vi "MintDAQ.vi"() -> ()   [LabVIEW 2016]
panel:
  in  "Freq":dbl=0.01
  in  "Amplitude 2":dbl
  in  "Amplitude":dbl
  in  "Freq":dbl=0.03
  in  "Write Rate":dbl=10.0 caption="dt"
  in  "Sampling Rate":dbl=40000.0
  in  "Buffer Size":i32=2000
  in  "Write":bool
  in  "?":T1(tab)=enum."Feedback"
  out "Autocollimator":dynamicdata(graph)=[{"t0"=timestamp(3581195496.5418625 s since 1904-01-01), "dt"=0.001, "Y"=[3.3748341722363353, 3.3776633625283514, 3.37797401320521, 3.3775669552805136, 3.3771035700077543, 3.3768751556826606, 3.376331438110049, 3.3762235118309984, 3.3790075255607244, 3.376298514761084, 3.3752552067778043, 3.376255087955073, 3.377024337467859, 3.377016265489406, 3.3768109764991143, 3.377772600659941, 3.3750167885038906, 3.3758342740501286, 3.3778386645680794, 3.377603931037596, 3.3773015918402085, 3.377296761916378, 3.377247926722811, 3.37593401556452, 3.3774822825090043, 3.3787107942105887, 3.376029554612824, 3.376047566746657, 3.376884514809987, 3.377298833130131, 3.3776098386367988, 3.37785651466396, 3.378069066780402, 3.3750767036010347, 3.377711191620555, 3.3788531793882703, 3.37852043613071, 3.378316912955789, 3.3779787548920632, 3.378261441737476, 3.3769786144398255, 3.3793285877009565, 3.378617996670578, 3.3764510415055766, 3.3768974602491557, 3.377733875773734, 3.377895089879731, 3.377746964024869, 3.378223767761222, 3.3771328113007395], "attributes"=variant("NI_ChannelName"=variant(string "Voltage_0 (Resampled)"), "NI_OriginalChannelName"=variant(string "Voltage_0"), "NI_UnitDescription"=variant(string "Volts"))}, {"t0"=timestamp(3581195496.5418625 s since 1904-01-01), "dt"=0.001, "Y"=[-2.0834369730605644, -2.0819321459746876, -2.0815308696350567, -2.082042347246933, -2.082466743846781, -2.082543042435832, -2.0827169780126265, -2.082885379693655, -2.080652839627904, -2.0814165804978457, -2.0830704383386687, -2.0833234560752936, -2.082983892721974, -2.0825139979157505, -2.082384163355347, -2.0813173776580993, -2.0827868935770524, -2.0834134790149905, -2.081433686965862, -2.081283686189381, -2.082151524207096, -2.082631712746277, -2.082526422863312, -2.082716175637639, -2.082090913848439, -2.080153207335917, -2.081799074668808, -2.0828669505009736, -2.082318511827896, -2.081803388234694, -2.081634121622563, -2.081400526460551, -2.080924953428108, -2.082794281679033, -2.0818087503052656, -2.080747192813816, -2.0808949294383616, -2.081554802023675, -2.081683750116512, -2.0816670043945638, -2.082051426671936, -2.0805717294034096, -2.079922992538738, -2.081701961823228, -2.082161220322588, -2.0816213289100975, -2.0813481659597706, -2.0809482340093424, -2.080058560613854, -2.08051520256095], "attributes"=variant("NI_ChannelName"=variant(string "Voltage_1 (Resampled)"), "NI_OriginalChannelName"=variant(string "Voltage_1"), "NI_UnitDescription"=variant(string "Volts"))}, {"t0"=timestamp(3581195496.5418625 s since 1904-01-01), "dt"=0.001, "Y"=[3.3920512615889953, 3.3949128153687473, 3.3955558463709457, 3.3949822866205603, 3.3944043177259724, 3.394248244026162, 3.3936132739947547, 3.393681652979987, 3.396403586319937, 3.3936103172767687, 3.3923165107027082, 3.393375095157017, 3.3944467686804276, 3.3945298904876613, 3.394206680532547, 3.395118492820506, 3.3923967067110294, 3.393226765021611, 3.395338486732797, 3.3951997197019326, 3.39470966390894, 3.3946116821482164, 3.3948381609352896, 3.393475746046146, 3.395065077505499, 3.3961215980661974, 3.393416269199552, 3.393221438439225, 3.394214058418473, 3.3947867354978474, 3.39488924630533, 3.3953627275736626, 3.3952376332484664, 3.3923657648357612, 3.395027357033787, 3.396204609534961, 3.396065231694474, 3.395684684123652, 3.3954015147584964, 3.395557924959077, 3.394371246663519, 3.3966569176530097, 3.3957795238341366, 3.3936416739636406, 3.394088238066653, 3.394798352283088, 3.3951686004824486, 3.3950579729554087, 3.3957615999214954, 3.394260081617193], "attributes"=variant("NI_ChannelName"=variant(string "Voltage_2 (Resampled)"), "NI_OriginalChannelName"=variant(string "Voltage_2"), "NI_UnitDescription"=variant(string "Volts"))}, {"t0"=timestamp(3581195496.5418625 s since 1904-01-01), "dt"=0.001, "Y"=[-4.704546009666462, -4.7034172877833775, -4.702890947722384, -4.703542130524446, -4.703923265813428, -4.704021939575232, -4.703693488617615, -4.704025410027072, -4.702148224679809, -4.702052254209579, -4.703534587738418, -4.703962279465137, -4.703948009827787, -4.703470533679648, -4.703105555572077, -4.702091625546342, -4.702915333730992, -4.70395319557882, -4.702507570272585, -4.702193733835325, -4.702668184050766, -4.703115504299192, -4.70302121431319, -4.702854412488044, -4.702826487004598, -4.700608325540924, -4.701635969066888, -4.703172652877774, -4.702721955144197, -4.702259181304256, -4.701769735302749, -4.702025515044418, -4.701073609491946, -4.702417864320141, -4.7023704513299, -4.701403031144604, -4.701670663349241, -4.702326994974521, -4.702301569985744, -4.702431205539657, -4.702584562170047, -4.701553485457985, -4.7001882132184445, -4.701730869681846, -4.702741761914817, -4.702399160645309, -4.702126691528818, -4.701683926466696, -4.701055859883961, -4.701163846839676], "attributes"=variant("NI_ChannelName"=variant(string "Voltage_3 (Resampled)"), "NI_OriginalChannelName"=variant(string "Voltage_3"), "NI_UnitDescription"=variant(string "Volts"))}]
  out "Interferometer":dynamicdata(graph)=[{"t0"=timestamp(3581195496.558861 s since 1904-01-01), "dt"=0.001, "Y"=[2.5754216942498864, 2.5742770760564575, 2.5752864512365665, 2.5755975336972146, 2.5764982112217156, 2.578020182032285, 2.5787188766928537, 2.578606033584902, 2.579588876887395, 2.5813718560222414, 2.5824290269137053, 2.5833332167546144, 2.584973605142916, 2.5865313596086486, 2.5867840974371945, 2.5874262183925896, 2.5883498262197056, 2.5884123817913567, 2.5880556867115208, 2.588476459648385, 2.5890038740074224, 2.590149046746964, 2.590527470266104, 2.5908797553704233, 2.5908021249703337, 2.5911027120717267, 2.5906961773826267, 2.5906389426042766, 2.5910755741104285, 2.5900107369525407, 2.588926999990385, 2.5871153489787506, 2.5858600365775013, 2.583231765079389, 2.5812393863898278, 2.57896258373196, 2.5773304396580587, 2.5750683414591737, 2.5742551919858183, 2.573192991734795, 2.5716328992763873, 2.57007305058364, 2.568897523403074, 2.5678238474894224, 2.5667978328234895, 2.567077680460652, 2.5667571629855264, 2.5660656544367746, 2.5656740216609126, 2.565405291450495], "attributes"=variant("NI_ChannelName"=variant(string "Voltage_0 (Resampled)"), "NI_OriginalChannelName"=variant(string "Voltage_0"), "NI_UnitDescription"=variant(string "Volts"))}, {"t0"=timestamp(3581195496.558861 s since 1904-01-01), "dt"=0.001, "Y"=[1.2793515572809446, 1.285498354667561, 1.285530841442421, 1.2866454157673533, 1.2869733309979952, 1.2847744418721374, 1.2839067641968223, 1.2851830164941183, 1.2832161133825573, 1.279361456728847, 1.2759169068675607, 1.2741532340418997, 1.2698705062094546, 1.2653216768729953, 1.264148206169354, 1.2617013703491549, 1.2588960289321576, 1.2573198229314126, 1.2586716578972597, 1.2561926025230898, 1.2542066243656944, 1.2503531667795282, 1.2484903412768558, 1.2474317144212412, 1.2463530521075994, 1.245232527609533, 1.245115686074537, 1.2441214009515857, 1.241348303995827, 1.2429377222051292, 1.2445254511305113, 1.2472626848196695, 1.2486097094585318, 1.2526354072563082, 1.2550193843337556, 1.2578768598051189, 1.2589034076207384, 1.2608772152092518, 1.2596400197842403, 1.2585228801854373, 1.259170816804813, 1.2607258750064372, 1.2614748165179137, 1.2624939000744886, 1.2631031863313682, 1.2612009551189116, 1.2603436196192965, 1.2612488256841587, 1.2611557894880032, 1.260442702752587], "attributes"=variant("NI_ChannelName"=variant(string "Voltage_1 (Resampled)"), "NI_OriginalChannelName"=variant(string "Voltage_1"), "NI_UnitDescription"=variant(string "Volts"))}]
  out "Interferometer Angle":dynamicdata(graph)=[{"t0"=timestamp(3581195496.558873 s since 1904-01-01), "dt"=0.001, "Y"=[1.279385757759777, 1.2855094923223165, 1.2855542287511086, 1.2867099167763918, 1.286990419041426, 1.2847176486281568, 1.2838809934099638, 1.2851425707064237, 1.283210596160443, 1.2793465166695555, 1.2759426302074155, 1.274074922473625, 1.2697739936917296, 1.2652325471941344, 1.2641815410790656, 1.2617045191057616, 1.258894905178912, 1.2572982837418094, 1.2586022040497762, 1.2561475450207342, 1.254186491101226, 1.250389088038898, 1.2484700760030873, 1.2474031281715254, 1.2462629746659435, 1.245226281697198, 1.2451530922726528, 1.244149659947579, 1.2413366614596872, 1.242918757455511, 1.2444992212566923, 1.247291337287777, 1.2486936729851912, 1.2527297438789293, 1.2550428009730812, 1.2578452899458512, 1.2588885866071604, 1.2608907125000104, 1.259678681049292, 1.2585387199133926, 1.259193832769137, 1.2606668939900645, 1.261480919713674, 1.2624981591153417, 1.2631580735971106, 1.2611901119476223, 1.2603383752109907, 1.2612189132061975, 1.2611199122397758, 1.2604627810897804], "attributes"=variant("NI_ChannelName"=variant(string "Voltage_1 (Resampled)"), "NI_OriginalChannelName"=variant(string "Voltage_1"), "NI_UnitDescription"=variant(string "Volts"))}]
  out "Autocollimator Angle":dynamicdata(graph)=[{"t0"=timestamp(3581195496.5418625 s since 1904-01-01), "dt"=0.001, "Y"=[-0.022423611113177477, -0.022450449019886524, -0.022855305793771385, -0.02263149446277486, -0.02248297326359854, -0.022581366665636312, -0.022435157319626368, -0.022722609422252498, -0.022636631966156725, -0.022470309983375715, -0.022181662951838568, -0.02226984750989989, -0.022657287009811056, -0.022770977196922157, -0.022615487010287802, -0.022533504364359788, -0.02254730770594651, -0.02264789077069858, -0.022758938900839965, -0.022867677268079374, -0.02263002876840118, -0.022511829189475786, -0.022868574094608053, -0.02278711992928183, -0.02289740781680684, -0.022594086661287316, -0.022582756534040693, -0.0223376458766495, -0.022537322747009748, -0.022734905524981537, -0.022467166045045037, -0.022786072671847766, -0.022281954078377453, -0.022464480051056616, -0.02254627646133278, -0.022559922703097778, -0.022801792854304097, -0.022570258329471692, -0.022651482643122833, -0.022487807540196154, -0.02261723046666237, -0.022564851290872264, -0.02226507168803021, -0.022338666744548097, -0.022360099135870695, -0.022198849876366833, -0.022457429594454455, -0.02249876198805851, -0.022809653060175253, -0.022224077364435976], "attributes"=variant("NI_ChannelName"=variant(string "Voltage_0 (Resampled)"), "NI_OriginalChannelName"=variant(string "Voltage_0"), "NI_UnitDescription"=variant(string "Volts"))}, {"t0"=timestamp(3581195496.5418625 s since 1904-01-01), "dt"=0.001, "Y"=[-3.407438558160998, -3.4079125742248393, -3.4077703512890656, -3.407959838855401, -3.407897265797124, -3.4079220295140447, -3.4072841963379528, -3.4074620940245945, -3.4079187381763134, -3.4068459952319516, -3.4066186655100212, -3.406828142701653, -3.4072510989553524, -3.407233556459601, -3.4069390278945857, -3.4070016417779705, -3.406198922977472, -3.406678419398217, -3.407387762350738, -3.4071922181277348, -3.406684063967491, -3.406631326487526, -3.406637564864018, -3.406191019434549, -3.406929141071579, -3.4065967898465237, -3.4058122827228736, -3.4063973950828714, -3.406517643799753, -3.406583380643447, -3.406175476469077, -3.406799151619011, -3.4061999314599913, -3.4055317218979666, -3.4067062404229853, -3.4068480112474, -3.4070131941908026, -3.4070066013790905, -3.4068023222572634, -3.406990179241895, -3.406688679595833, -3.4072419272150936, -3.4063615605901414, -3.4060575146095364, -3.4067500052994264, -3.407007580810114, -3.407006760653448, -3.4069511985991308, -3.407278167995152, -3.406869057652937], "attributes"=variant("NI_ChannelName"=variant(string "Voltage_3 (Resampled)"), "NI_OriginalChannelName"=variant(string "Voltage_3"), "NI_UnitDescription"=variant(string "Volts"))}]
  in  "PID Input":bool
  out "Feedback":dynamicdata(graph)=[{"t0"=timestamp(3581195496.541873 s since 1904-01-01), "dt"=0.001, "Y"=[3.00026509800258, 3.000265622029558, 3.000266145122005, 3.000266667280689, 3.0002671885063976, 3.0002677088000196, 3.0002682281622066, 3.0002687465938225, 3.0002692640955293, 3.0002697806681904, 3.0002702963124177, 3.0002708110293135, 3.000271324819598, 3.0002718376838167, 3.0002723496228616, 3.0002728606376117, 3.0002733707288565, 3.0002738798973905, 3.0002743881440366, 3.0002748954694245, 3.000275401874374, 3.0002759073596024, 3.000276411925802, 3.0002769155738234, 3.000277418304465, 3.000277920118473, 3.000278421016645, 3.0002789209996665, 3.000279420068413, 3.000279918223621, 3.000280415466136, 3.000280911796708, 3.0002814072159985, 3.000281901724924, 3.0002823953243563, 3.0002828880149255, 3.0002833797974575, 3.000283870672715, 3.000284360641512, 3.0002848497046695, 3.0002853378629677, 3.0002858251169577, 3.0002863114674496, 3.0002867969153555, 3.000287281461401, 3.0002877651063673, 3.0002882478508788, 3.0002887296956446, 3.000289210641672, 3.000289690689525], "attributes"=variant("NI_ChannelName"=variant(string "Voltage_0 (Resampled)"), "NI_OriginalChannelName"=variant(string "Voltage_0"), "NI_UnitDescription"=variant(string "Volts"))}, {"t0"=timestamp(3581195496.541873 s since 1904-01-01), "dt"=0.001, "Y"=[2.981366981682563, 2.981681201423416, 2.9818233878908376, 2.9820361021397925, 2.982147718637047, 2.9815284317106263, 2.9815931630449275, 2.981874007612584, 2.982072168553749, 2.982184440496617, 2.981801962365537, 2.9817788984235003, 2.9818820278062894, 2.9819765819480586, 2.9818494719532476, 2.9813457380983692, 2.981733384334563, 2.9818258894115055, 2.9819692934268147, 2.9819237031683543, 2.9817359774003815, 2.9817910727751586, 2.9818370933873006, 2.981962335777197, 2.981527236704181, 2.9816001051787917, 2.981835414551896, 2.9818779209902457, 2.9820196614799537, 2.981539067398664, 2.981673579371675, 2.9818896310670353, 2.9818991799823187, 2.9818536008663785, 2.9816737333564594, 2.9818386632493694, 2.981896088828551, 2.981933594686985, 2.982082140033311, 2.981901742387895, 2.981871599760998, 2.9818306093229183, 2.982084066239377, 2.9824729167034496, 2.9817400167741246, 2.981732127877782, 2.9818772880175404, 2.982147999367483, 2.9821822707943397, 2.9814515305916562], "attributes"=variant("NI_ChannelName"=variant(string "Voltage_4 (Resampled)"), "NI_OriginalChannelName"=variant(string "Voltage_4"), "NI_UnitDescription"=variant(string "Volts"))}, {"t0"=timestamp(3581195496.541873 s since 1904-01-01), "dt"=0.001, "Y"=[-0.017250004454718724, -0.017271911011308747, -0.017583460962599072, -0.01740578906570031, -0.017292778036316393, -0.01736623340481054, -0.01726155536138694, -0.01747654623861962, -0.01741169197440696, -0.01727766103186276, -0.01706353295485361, -0.017134370003069645, -0.017431043722846137, -0.01752071106259731, -0.017397237704261295, -0.017332737135086707, -0.017343574930380443, -0.017418952713191365, -0.017507720396789085, -0.017590212842876415, -0.017403856881993505, -0.017318384903411907, -0.017596261548920765, -0.01753216057808684, -0.01761251342378257, -0.017381662567338235, -0.01736747494467825, -0.017185319404453853, -0.01733902310388046, -0.01748491353820703, -0.01728461356031098, -0.01752528372507638, -0.017139163870553406, -0.017281951077263914, -0.017345862434854826, -0.017355253899807296, -0.01753641319253484, -0.017358121559445872, -0.01742772100948116, -0.01729449832409784, -0.017397030426622936, -0.017356070614192, -0.017124117152675707, -0.01718638219487926, -0.01719766855612775, -0.017076674961508716, -0.017274466489494246, -0.017309589109020487, -0.017541464502398, -0.017095535812710817], "attributes"=variant("NI_ChannelName"=variant(string "Voltage_0 (Resampled)"), "NI_OriginalChannelName"=variant(string "Voltage_0"), "NI_UnitDescription"=variant(string "Volts"))}, {"t0"=timestamp(3581195496.508873 s since 1904-01-01), "dt"=0.001, "Y"=[0.0004357490019484657, 0.000436304324749317, 0.000437144367764738, 0.0004369795161564038, 0.00043645808160936426, 0.00043622096671427256, 0.00043576804521063906, 0.0004353960409446345, 0.00043499361434182383, 0.00043471696541827086, 0.0004344487571499159, 0.0004335807529681782, 0.00043330642598976175, 0.00043267191943170024, 0.0004333933484677321, 0.00043378996654489617, 0.00043455761747122554, 0.0004338058658537336, 0.0004340102119713781, 0.0004331556772335303, 0.00043186317343093535, 0.000430894051508061, 0.00043022501090551044, 0.0004292892435043405, 0.0004278637104570139, 0.00042699720914467264, 0.00042610956223811195, 0.00042504241551064346, 0.00042414937586284337, 0.0004233540483542753, 0.00042247332209719216, 0.00042258394079659544, 0.0004233766184508551, 0.0004240055209919068, 0.0004241671191234005, 0.00042435123794270135, 0.00042439237774010476, 0.0004234363160699178, 0.0004230036139324838, 0.00042290515991437894, 0.0004227196924963413, 0.000421623421036249, 0.0004211476728621625, 0.0004207800354503167, 0.00042104262157576595, 0.00042091638647550055, 0.00042107031652104197, 0.00042242861169140063, 0.00042348952497543404, 0.0004248686467799726], "attributes"=variant("NI_ChannelName"=variant(string "Voltage_1 (Resampled)"), "NI_OriginalChannelName"=variant(string "Voltage_1"), "NI_UnitDescription"=variant(string "Volts"))}]
  in  "Offset 1":dbl=3.0
  in  "Offset 2":dbl=3.0
  in  "AC Setpoint":dbl=0.0128
  in  "Gain":dbl
  in  "I term":dbl=0.014
  in  "Reset Button":bool
  in  "D term":dbl=90.0
  in  "Int Setpoint":dbl=0.0011
  # "Swing\nInjection"
  # "Torsion\nInjectio"
  # "Interferometer"
  # "Autocollimator"
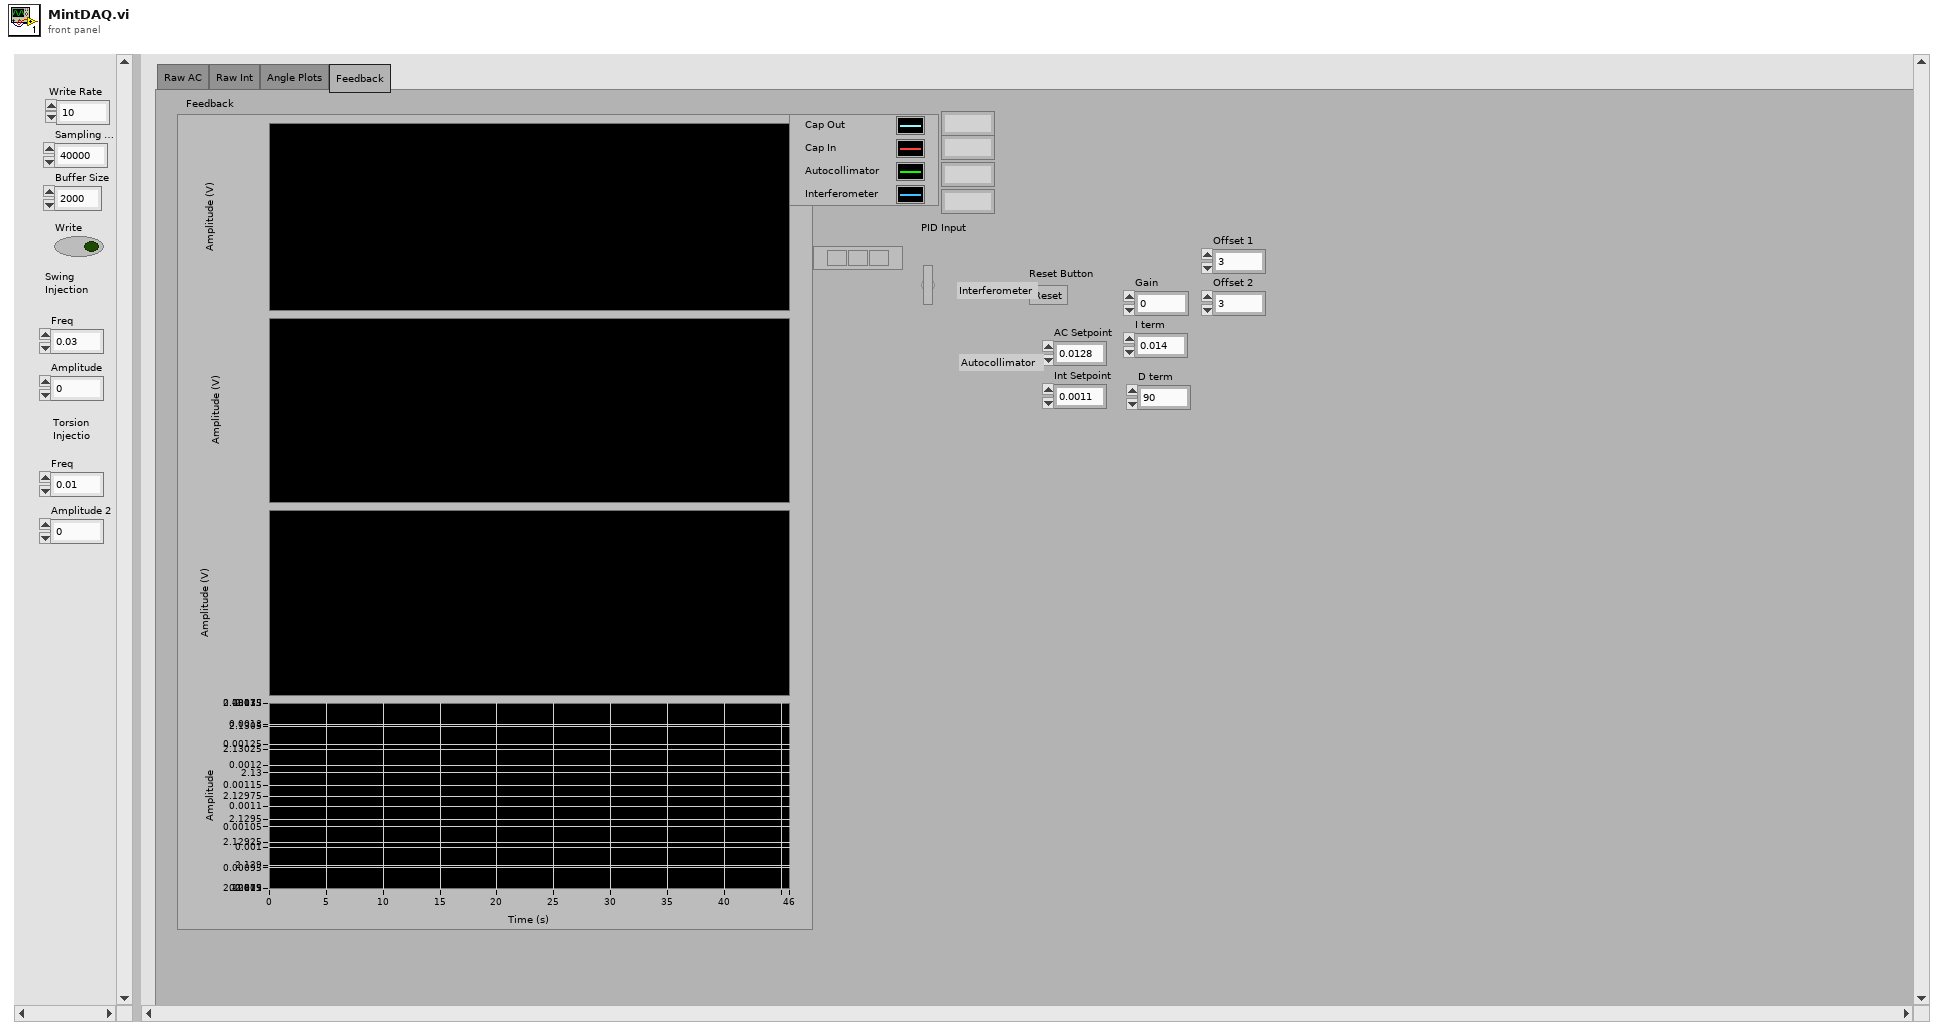
[diagram p1: front panel]
types:
  T1 = enum32{"Raw AC", "Raw Int", "Angle Plots", "Feedback"}
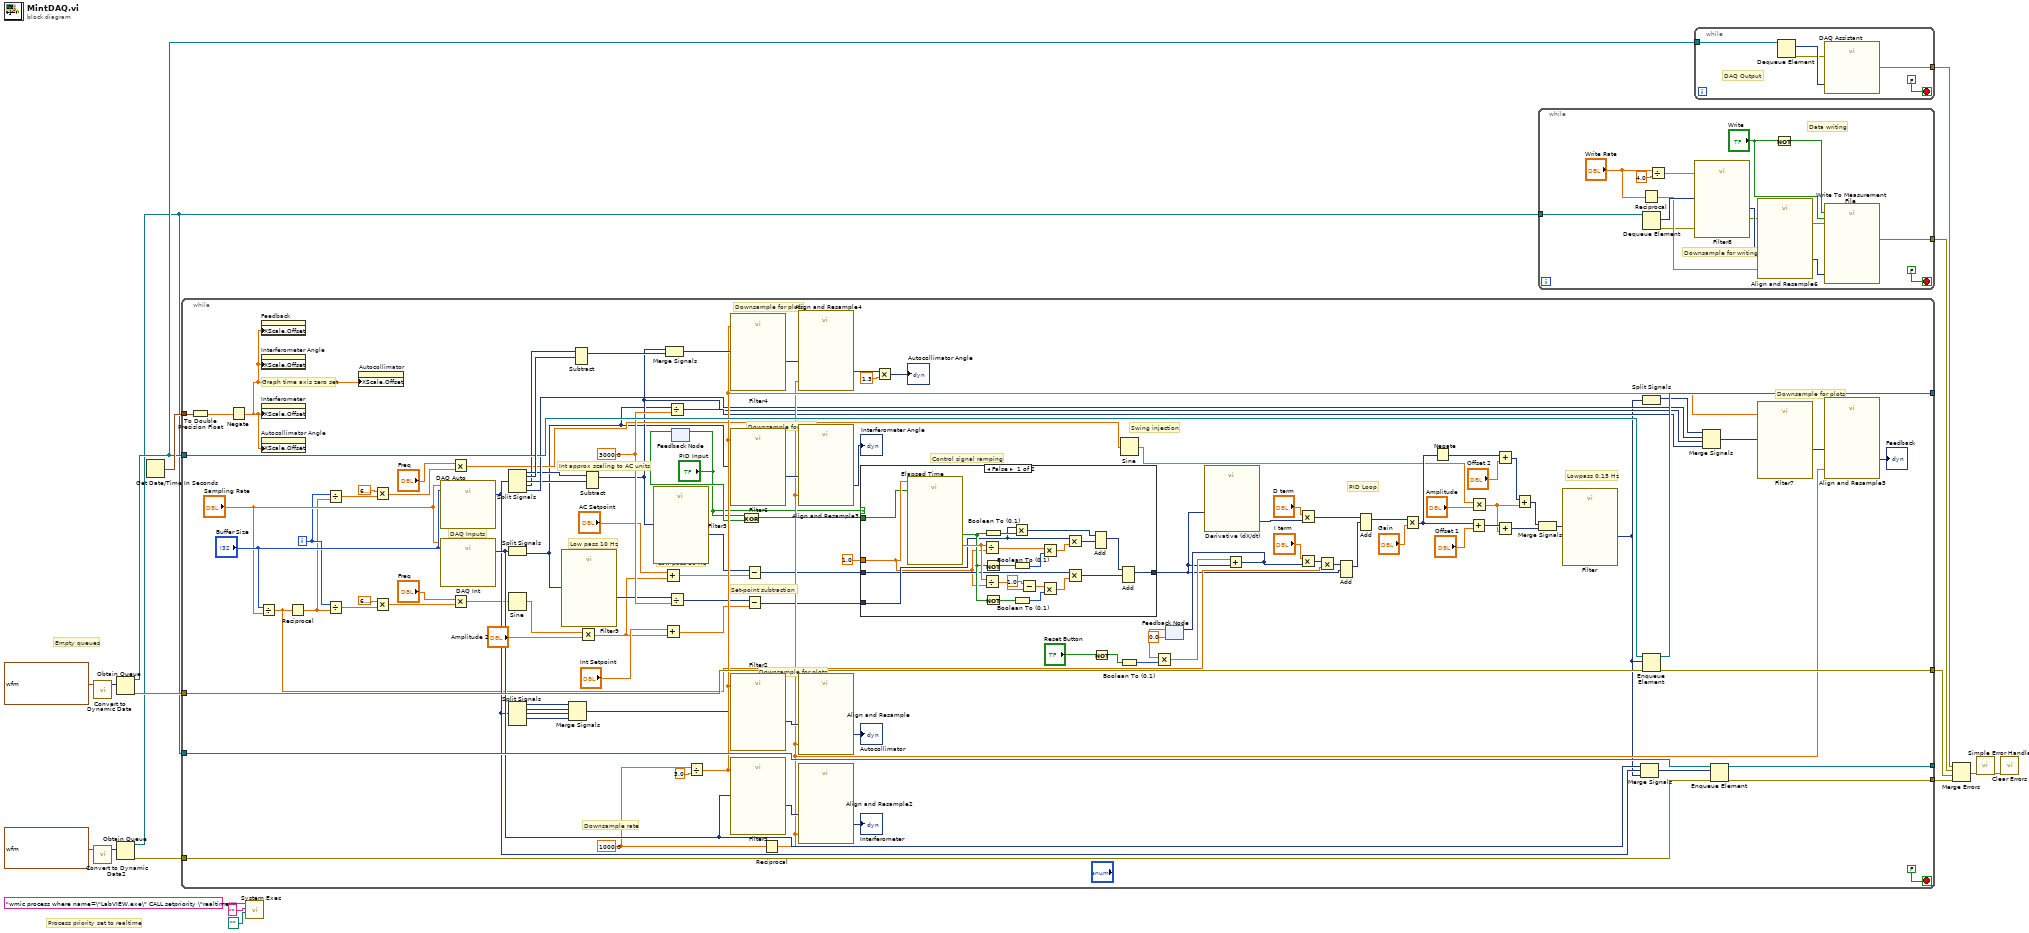
[diagram p0: block diagram]
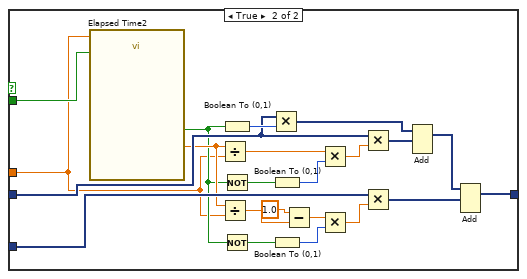
[diagram p2: hidden frame]
diagram:
  # "Empty queues"
  # "Process priority set to realtime"
  n1 = call "Convert to Dynamic Data"("Waveform"=waveform(dbl) {"t0"=timestamp(0 s since 1904-01-01), "dt"=1.0, "Y"=[]}) -> ("Dynamic Data Type"=w16:dynamicdata)  [unwired: 3 in]
  n2 = call "Convert to Dynamic Data2"("Waveform"=waveform(dbl) {"t0"=timestamp(0 s since 1904-01-01), "dt"=1.0, "Y"=[]}) -> ("Dynamic Data Type"=w14:dynamicdata)  [unwired: 3 in]
  n3 = Obtain Queue(element data type=w16) -> (queue out=w11:refnum<queue>, error out=w13:errorcluster)  [unwired: 4 in, 1 out]
  n4 = Obtain Queue(element data type=w14) -> (queue out=w10:refnum<queue>, error out=w12:errorcluster)  [unwired: 4 in, 1 out]
  n5 = Get Date/Time In Seconds() -> (seconds since 1Jan1904=w18:timestamp)
  n6 = while {
    tunnel: w18 -> [w127]
    tunnel: w11 -> [w123]
    tunnel: [w122] -> _
    tunnel: w10 -> [w106]
    tunnel: [w105] -> _
    tunnel: w13 -> [w104]
    tunnel: w12 -> [w103]
    tunnel: [w102] -> w8
    tunnel: [w101] -> w9
    i -> [w41]
    stop <- FALSE stop-if-true
    w82 = 3000.0 ("y")
    w86 = 1000.0 ("dt")
    # "Downsample for plots"
    # "Lowpass 0.15 Hz"
    # "PID Loop"
    # "Control signal ramping"
    # "Swing injection"
    # "Downsample rate"
    # "Downsample for plots"
    # "Downsample for plots"
    # "Downsample for plots"
    # "Int approx scaling to AC units"
    # "Set-point subtraction"
    # "Low pass 10 Hz"
    # "Low pass 10 Hz"
    # "DAQ Inputs"
    # "Graph time axis zero set"
    n7 = To Double Precision Float(number=w127) -> (double precision float=w126:dbl)
    n8 = Negate(x=w126) -> (-x=w124:dbl)
    n9 = Divide(x="Buffer Size", y="Sampling Rate") -> (x/y=w46:dbl)
    n10 = property on="Feedback" class="WFChart (strict)"("XScale.Offset"=w124) -> ()  [unwired: 2 in, 2 out]
    n11 = property on="Interferometer Angle" class="WFChart (strict)"("XScale.Offset"=w124) -> ()  [unwired: 2 in, 2 out]
    n12 = property on="Interferometer" class="WFChart (strict)"("XScale.Offset"=w124) -> ()  [unwired: 2 in, 2 out]
    n13 = property on="Autocollimator Angle" class="WFChart (strict)"("XScale.Offset"=w124) -> ()  [unwired: 2 in, 2 out]
    n14 = Reciprocal(x=w46) -> (1/x=w40:dbl)
    n15 = Divide(x=w41, y=w40) -> (x/y=w57:dbl)
    n16 = Divide(x=w41, y=w40) -> (x/y=w42:dbl)
    n17 = property on="Autocollimator" class="WFChart (strict)"("XScale.Offset"=w124) -> ()  [unwired: 2 in, 2 out]
    n18 = Multiply(x=6.283185307179586, y=w57) -> (x*y=w56:dbl)
    n19 = Multiply(x=6.283185307179586, y=w42) -> (x*y=w43:dbl)
    n20 = call "DAQ Auto"("rate"="Sampling Rate", "number of samples"="Buffer Size") -> ("data"=w64:dynamicdata)  [unwired: 14 in, 3 out]
    n21 = call "DAQ Int"("rate"="Sampling Rate", "number of samples"="Buffer Size") -> ("data"=w92:dynamicdata)  [unwired: 14 in, 3 out]
    n22 = Multiply(x="Freq", y=w56) -> (x*y=w54:dbl)
    n23 = Multiply(x="Freq", y=w43) -> (x*y=w44:dbl)
    n24 = Split Signals(w64) -> (w78:dynamicdata, w125:dynamicdata, w77:dynamicdata, w76:dynamicdata, w84:dynamicdata)  [unwired: 5 in]
    n25 = Split Signals(w92) -> (w35:dynamicdata)  [unwired: 2 in, 1 out]
    n26 = Sine(x=w44) -> (sin(x)=w45:dbl)
    n27 = Split Signals(w64) -> (w69:dynamicdata, w68:dynamicdata, w67:dynamicdata, w66:dynamicdata)  [unwired: 5 in, 1 out]
    n28 = call "Filter9"("Signal"=w35) -> ("Filtered Signal"=w34:dynamicdata)  [unwired: 9 in, 1 out]
    n29 = Merge Signals(w69, w68, w67, w66) -> (w65:dynamicdata)
    n30 = Subtract(1:w125, 2:w76) -> (0:w75:dynamicdata)  [unwired: 1 in, 1 out]
    n31 = Multiply(x=w45, y="Amplitude 2") -> (x*y=w28:dbl)
    n32 = Subtract(1:w77, 2:w78) -> (0:w36:dynamicdata)  [unwired: 1 in, 1 out]
    n33 = call "Filter3"("Signal"=w36) -> ("Filtered Signal"=w30:dynamicdata)  [unwired: 9 in, 1 out]
    n34 = Add(x="AC Setpoint", y=w28) -> (x+y=w31:dbl)
    n35 = Add(x="Int Setpoint", y=w28) -> (x+y=w33:dbl)
    n36 = Merge Signals(w36, w75) -> (w94:dynamicdata)
    n37 = Divide(x=w35, y=w82) -> (x/y=w83:dynamicdata)
    n38 = Divide(x=w34, y=w82) -> (x/y=w32:dynamicdata)
    n39 = feedback #1() -> (w25:bool)  [unwired: 1 in]
    n40 = feedback-in #1("PID Input") -> ()
    n41 = Divide(x=w86, y=3.0) -> (x/y=w87:dbl)
    n42 = call "Filter4"("Lower Cut-Off"=w87, "Signal"=w94) -> ("Filtered Signal"=w93:dynamicdata)  [unwired: 8 in, 1 out]
    n43 = call "Filter6"("Lower Cut-Off"=w87, "Signal"=w35) -> ("Filtered Signal"=w90:dynamicdata)  [unwired: 8 in, 1 out]
    n44 = call "Filter2"("Lower Cut-Off"=w87, "Signal"=w65) -> ("Filtered Signal"=w95:dynamicdata)  [unwired: 8 in, 1 out]
    n45 = call "Filter5"("Lower Cut-Off"=w87, "Signal"=w92) -> ("Filtered Signal"=w91:dynamicdata)  [unwired: 8 in, 1 out]
    n46 = Exclusive Or(1:w25, 2:"PID Input") -> (0:w24:bool)
    n47 = Subtract(x=w30, y=w31) -> (x-y=w22:dynamicdata)
    n48 = Subtract(x=w32, y=w33) -> (x-y=w21:dynamicdata)
    n49 = Reciprocal(x=w86) -> (1/x=w85:dbl)
    n50 = call "Align and Resample4"("dt"=w85, "Signals"=w93) -> ("Resampled Signals"=w80:dynamicdata)  [unwired: 7 in, 2 out]
    n51 = call "Align and Resample3"("dt"=w85, "Signals"=w90) -> ("Resampled Signals"=→"Interferometer Angle":dynamicdata)  [unwired: 7 in, 2 out]
    n52 = call "Align and Resample"("dt"=w85, "Signals"=w95) -> ("Resampled Signals"=→"Autocollimator":dynamicdata)  [unwired: 7 in, 2 out]
    n53 = call "Align and Resample2"("dt"=w85, "Signals"=w91) -> ("Resampled Signals"=→"Interferometer":dynamicdata)  [unwired: 7 in, 2 out]
    n54 = case shown="False" "PID Input" {
      tunnel: w21 -> [w133 w161]
      tunnel: w22 -> [w132 w166]
      tunnel: [w129 w152] -> w19
      tunnel: w24 -> [w130 w164]
      tunnel: 1.0 ("y") -> [w131 w151]
      frame False {
        n55 = call "Elapsed Time"("Time Target (s)"=w131, "Reset"=w130) -> ("Elapsed Time (s)"=w138:dbl, "Time has Elapsed"=w136:bool)  [unwired: 10 in, 6 out]
        n56 = Divide(x=w138, y=w131) -> (x/y=w144:dbl)
        n57 = Divide(x=w138, y=w131) -> (x/y=w140:dbl)
        n58 = Boolean To (0,1)(Boolean=w136) -> (0, 1=w150:i16)
        n59 = Not(x=w136) -> (.not. x?=w145:bool)
        n60 = Not(x=w136) -> (.not. x?=w137:bool)
        n61 = Multiply(x=w133, y=w150) -> (x*y=w148:dynamicdata)
        n62 = Boolean To (0,1)(Boolean=w145) -> (0, 1=w147:i16)
        n63 = Boolean To (0,1)(Boolean=w137) -> (0, 1=w143:i16)
        n64 = Subtract(x=1.0, y=w140) -> (x-y=w139:dbl)
        n65 = Multiply(x=w144, y=w147) -> (x*y=w146:dbl)
        n66 = Multiply(x=w139, y=w143) -> (x*y=w142:dbl)
        n67 = Multiply(x=w133, y=w146) -> (x*y=w149:dynamicdata)
        n68 = Multiply(x=w132, y=w142) -> (x*y=w135:dynamicdata)
        n69 = Add(1:w149, 2:w148) -> (0:w134:dynamicdata)  [unwired: 1 in, 1 out]
        n70 = Add(1:w135, 2:w134) -> (0:w129:dynamicdata)  [unwired: 1 in, 1 out]
      }
      frame True {
        n71 = call "Elapsed Time2"("Time Target (s)"=w151, "Reset"=w164) -> ("Elapsed Time (s)"=w157:dbl, "Time has Elapsed"=w155:bool)  [unwired: 10 in, 6 out]
        n72 = Divide(x=w157, y=w151) -> (x/y=w165:dbl)
        n73 = Divide(x=w157, y=w151) -> (x/y=w159:dbl)
        n74 = Boolean To (0,1)(Boolean=w155) -> (0, 1=w172:i16)
        n75 = Not(x=w155) -> (.not. x?=w167:bool)
        n76 = Not(x=w155) -> (.not. x?=w156:bool)
        n77 = Multiply(x=w166, y=w172) -> (x*y=w170:dynamicdata)
        n78 = Boolean To (0,1)(Boolean=w167) -> (0, 1=w169:i16)
        n79 = Boolean To (0,1)(Boolean=w156) -> (0, 1=w163:i16)
        n80 = Subtract(x=1.0, y=w159) -> (x-y=w158:dbl)
        n81 = Multiply(x=w165, y=w169) -> (x*y=w168:dbl)
        n82 = Multiply(x=w158, y=w163) -> (x*y=w162:dbl)
        n83 = Multiply(x=w166, y=w168) -> (x*y=w171:dynamicdata)
        n84 = Multiply(x=w161, y=w162) -> (x*y=w154:dynamicdata)
        n85 = Add(1:w171, 2:w170) -> (0:w153:dynamicdata)  [unwired: 1 in, 1 out]
        n86 = Add(1:w154, 2:w153) -> (0:w152:dynamicdata)  [unwired: 1 in, 1 out]
      }
    }
    n87 = Multiply(x=w80, y=1.3) -> (x*y=→"Autocollimator Angle":dynamicdata)
    n88 = Not(x="Reset Button") -> (.not. x?=w117:bool)
    n89 = Boolean To (0,1)(Boolean=w117) -> (0, 1=w71:i16)
    n90 = Sine(x=w54) -> (sin(x)=w53:dbl)
    n91 = feedback #2(0.0) -> (w73:dbl)
    n92 = Multiply(x=w73, y=w71) -> (x*y=w72:dbl)
    n93 = call "Derivative (dX/dt)"("Signals"=w19) -> ("Result"=w116:dynamicdata)  [unwired: 5 in, 1 out]
    n94 = Add(x=w72, y=w19) -> (x+y=w70:dynamicdata)
    n95 = feedback-in #2(w70) -> ()
    n96 = Multiply(x="D term", y=w116) -> (x*y=w114:dynamicdata)
    n97 = Multiply(x="I term", y=w70) -> (x*y=w63:dynamicdata)
    n98 = Multiply(x=w63, y=w46) -> (x*y=w61:dynamicdata)
    n99 = Add(1:w19, 2:w61) -> (0:w113:dynamicdata)  [unwired: 1 in, 1 out]
    n100 = Add(1:w113, 2:w114) -> (0:w112:dynamicdata)  [unwired: 1 in, 1 out]
    n101 = Multiply(x=w112, y="Gain") -> (x*y=w108:dynamicdata)
    n102 = Negate(x=w108) -> (-x=w109:dynamicdata)
    n103 = Add(x=w108, y="Offset 1") -> (x+y=w51:dynamicdata)
    n104 = Multiply(x=w53, y="Amplitude") -> (x*y=w47:dbl)
    n105 = Add(x=w109, y="Offset 2") -> (x+y=w49:dynamicdata)
    n106 = Add(x=w51, y=w47) -> (x+y=w50:dynamicdata)
    n107 = Add(x=w49, y=w47) -> (x+y=w48:dynamicdata)
    n108 = Merge Signals(w48, w50) -> (w27:dynamicdata)
    n109 = call "Filter"("Signal"=w27) -> ("Filtered Signal"=w26:dynamicdata)  [unwired: 9 in, 1 out]
    n110 = Merge Signals(w92, w64, w26) -> (w107:dynamicdata)
    n111 = Split Signals(w26) -> (w121:dynamicdata)  [unwired: 2 in, 1 out]
    n112 = Enqueue Element(queue=w123, element=w26, error in (no error)=w104) -> (queue out=w122:refnum<queue>, error out=w102:errorcluster)  [unwired: 1 in, 1 out]
    n113 = Merge Signals(w121, w84, w36, w83) -> (w89:dynamicdata)
    n114 = Enqueue Element(queue=w106, element=w107, error in (no error)=w103) -> (queue out=w105:refnum<queue>, error out=w101:errorcluster)  [unwired: 1 in, 1 out]
    n115 = call "Filter7"("Lower Cut-Off"=w87, "Signal"=w89) -> ("Filtered Signal"=w88:dynamicdata)  [unwired: 8 in, 1 out]
    n116 = call "Align and Resample5"("dt"=w85, "Signals"=w88) -> ("Resampled Signals"=→"Feedback":dynamicdata)  [unwired: 7 in, 2 out]
  }
  n117 = call <vilib>:"System Exec.vi"("working directory"=path "", "standard input"="", "command line"="wmic process where name=\"LabVIEW.exe\" CALL setpriority \"realtime\"") -> ()  [unwired: 5 in, 4 out]
  n118 = while {
    tunnel: w10 -> [w186]
    tunnel: [w173] -> w5
    stop <- FALSE stop-if-true
    # "Downsample for writing"
    # "Data writing"
    n119 = Reciprocal(x="Write Rate") -> (1/x=w182:dbl)
    n120 = Dequeue Element(queue=w186) -> (element=w184:dynamicdata, error out=w176:errorcluster)  [unwired: 2 in, 2 out]
    n121 = Divide(x="Write Rate", y=4.0) -> (x/y=w181:dbl)
    n122 = call "Filter8"("error in (no error)"=w176, "Lower Cut-Off"=w181, "Signal"=w184) -> ("error out"=w175:errorcluster, "Filtered Signal"=w185:dynamicdata)  [unwired: 7 in]
    n123 = call "Align and Resample6"("dt"=w182, "error in (no error)"=w175, "Signals"=w185) -> ("error out"=w174:errorcluster, "Resampled Signals"=w183:dynamicdata)  [unwired: 6 in, 1 out]
    n124 = Not(x="Write") -> (.not. x?=w177:bool)
    n125 = call "Write To Measurement File"("Signals"=w183, "Reset"=w177, "Enable"="Write", "error in (no error)"=w174) -> ("error out"=w173:errorcluster)  [unwired: 13 in, 2 out]
  }
  n126 = while {
    tunnel: w11 -> [w191]
    tunnel: [w188] -> w4
    stop <- FALSE stop-if-true
    # "DAQ Output"
    n127 = Dequeue Element(queue=w191) -> (element=w190:dynamicdata, error out=w189:errorcluster)  [unwired: 2 in, 2 out]
    n128 = call "DAQ Assistant"("data"=w190, "error in"=w189) -> ("error out"=w188:errorcluster)  [unwired: 16 in, 1 out]
  }
  n129 = Merge Errors(w4, w5, w8, w9) -> (w6:errorcluster)
  n130 = call <vilib>:"Simple Error Handler.vi"("error in (no error)"=w6) -> ("error out"=w7:errorcluster)  [unwired: 4 in, 4 out]
  n131 = call <vilib>:"Clear Errors.vi"("error in (no error)"=w7) -> ()  [unwired: 5 in, 2 out]
